vi "Write Control Data to Config File - Num.vi"(8 "error in (no error)":errorcluster, 10 "Num Controls":refnum<vi>[](array[refnum]), 11 "Config File Path":path) -> (0 "error out":errorcluster)   [LabVIEW 2018]
uses:
  <vilib>/Utility/config.llb/Write Key (Double).vi
  <vilib>/Utility/config.llb/NI_LVConfig.lvlib
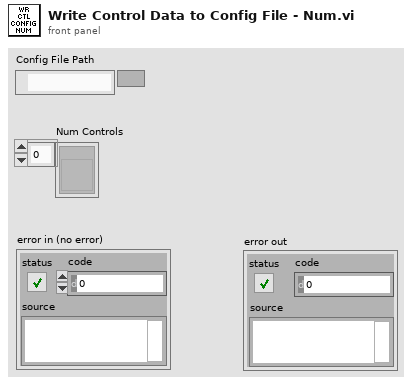
[diagram p1: front panel]
types:
  T1 = typedef "NI_LVConfig.lvlib/Config Data RefNum.ctl" = refnum<k1>
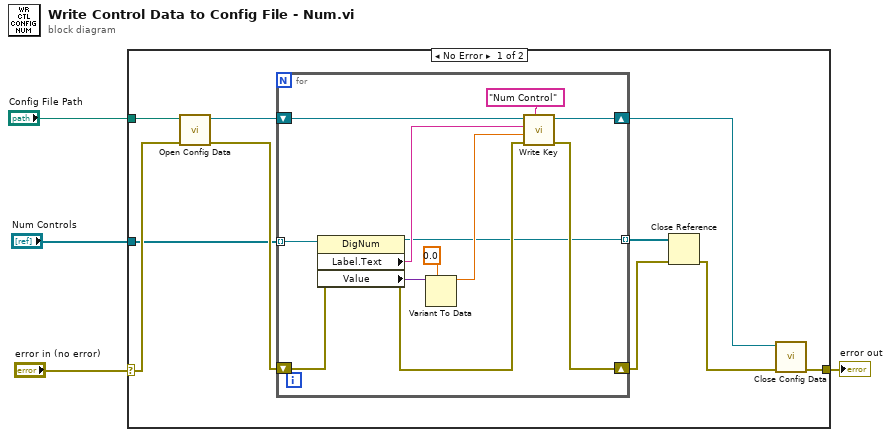
[diagram p0: block diagram]
diagram:
  n1 = case shown="No Error" "error in (no error)" {
    selector: "error in (no error)" -> [w11 w27]
    tunnel: "Config File Path" -> [w12 _]
    tunnel: "Num Controls" -> [w10 _]
    tunnel: [w5 w27] -> w1
    frame No Error {
      n2 = call <vilib>:"Open Config Data.vi"("error in (no error)"=w11, "configuration file path"=w12) -> ("error out"=w13:errorcluster, "refnum"=w14:T1)  [unwired: 7 in, 1 out]
      n3 = for {
        shift-right: [w24] -> w8
        shift-left: w14 -> [w25]
        shift-right: [w23] -> w7
        shift-left: w13 -> [w21]
        tunnel: w10 -> [w22] mode=indexing
        tunnel: [w15] -> w9 mode=indexing
        n4 = property class="DigNum"(reference=w22, error in=w21) -> (reference out=w15:refnum<vi>, error out=w16:errorcluster, "Label.Text"=w20:string, "Value"=w19:variant)
        n5 = Variant To Data(type=0.0, Variant=w19) -> (data=w17:dbl)  [unwired: 1 in, 1 out]
        n6 = call-poly <vilib>:"Write Key.vi"("section"="Num Control", "error in (no error)"=w16, "value"=w17, "key"=w20, "refnum"=w25) -> ("error out"=w23:errorcluster, "refnum out"=w24:T1)  [unwired: 3 in, 2 out]
      }
      n7 = Close Reference(reference=w9, error in (no error)=w7) -> (error out=w6:errorcluster)
      n8 = call <vilib>:"Close Config Data.vi"("error in (no error)"=w6, "refnum"=w8) -> ("error out"=w5:errorcluster)  [unwired: 8 in, 1 out]
    }
    frame Error {
    }
  }
  "error out" <- w1
